vi "Periodic Tasks.vi"(8 "error in":errorcluster) -> ()   [LabVIEW 2017]
doc: "This VI runs in parallel to other robot code. It can contain as many user-defined periodic loops as you need. These can carry out PID or other sorts of timed response."
uses:
  <vilib>/Rock Robotics/Network Tables/NT Read String.vi
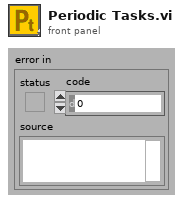
[diagram p1: front panel]
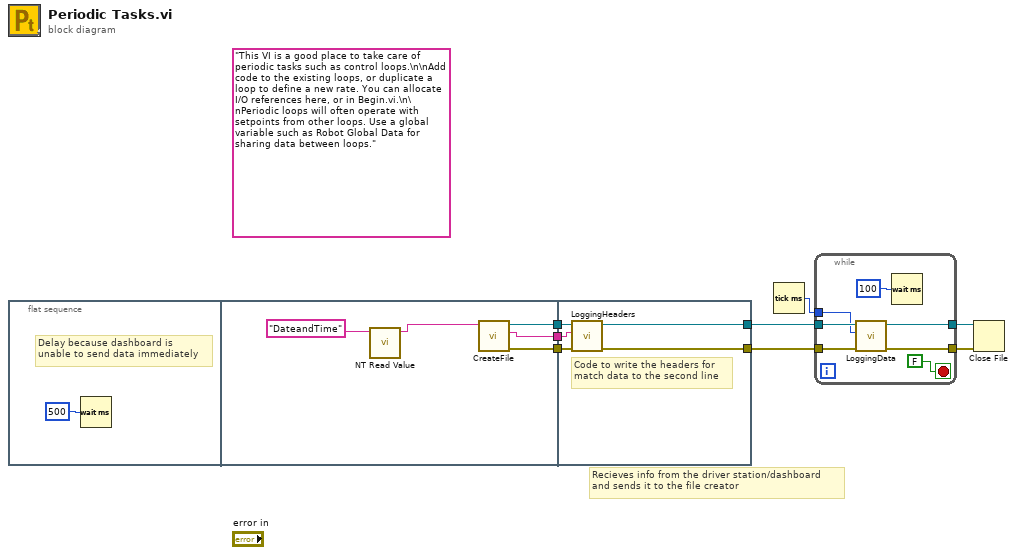
[diagram p0: block diagram]
diagram:
  (unwired) "This VI is a good place to take care of periodic tasks such as control loops.\n\nAdd code to the existing loops, or duplicate a loop to define a new rate. You can allocate I/O references here, or in Begin.vi.\n\nPeriodic loops will often operate with setpoints from other loops. Use a global variable such as Robot Global Data for sharing data between loops."
  # "Recieves info from the driver station/dashboard\nand sends it to the file creator"
  n1 = flat-sequence {
    tunnel: [w14] -> w7
    tunnel: [w12] -> w8
    tunnel: [w13] -> w6
    tunnel: w8 -> [w17]
    tunnel: w7 -> [w18]
    tunnel: w6 -> [w19]
    tunnel: [w16] -> w4
    tunnel: [w15] -> w3
    frame #0 {
      # "Delay because dashboard is \nunable to send data immediately"
      n2 = Wait (ms)(milliseconds to wait=u32 500) -> ()  [unwired: 1 out]
    }
    frame #1 {
      n3 = call-poly <vilib>:"NT Read Value.vi"("Name"="DateandTime") -> ("String"=w10:string)  [unwired: 9 in, 1 out]
      n4 = call "CreateFile.vi"("Date/time"=w10) -> ("error out"=w13:errorcluster, "Date/Time"=w12:string, "Byte Stream File out"=w14:refnum<file>)  [unwired: 8 in]
    }
    frame #2 {
      # "Code to write the headers for \nmatch data to the second line"
      n5 = call "LoggingHeaders.vi"("error in"=w19, "Date and Time"=w17, "refnum in"=w18) -> ("error out"=w15:errorcluster, "refnum out"=w16:refnum<file>)  [unwired: 7 in]
    }
  }
  n6 = Tick Count (ms)() -> (millisecond timer value=w5:u32)
  n7 = while {
    tunnel: w5 -> [w22]
    tunnel: w4 -> [w24]
    tunnel: w3 -> [w23]
    tunnel: [w21] -> w2
    tunnel: [w20] -> w1
    stop <- FALSE stop-if-true
    n8 = call "LoggingData.vi"("error in (no error)"=w23, "Start time"=w22, "Refmum"=w24) -> ("error out"=w20:errorcluster, "Byte Stream File out"=w21:refnum<file>)  [unwired: 7 in]
    n9 = Wait (ms)(milliseconds to wait=u32 100) -> ()  [unwired: 1 out]
  }
  n10 = Close File(refnum=w2, error in=w1) -> ()  [unwired: 2 out]
